vi "Get init instructions.vi"(8 "error in (no error)":errorcluster, 11 "Motor in":refnum<class "Motor.lvclass">) -> (0 "error out":errorcluster, 1 "name":string, 2 "init instructions":string[](array[string]), 3 "Motor out":refnum<class "Motor.lvclass">)   [LabVIEW 2018, in "Motor.lvclass"]
uses:
  Motor.lvclass
  Motor.lvclass/Motor.ctl
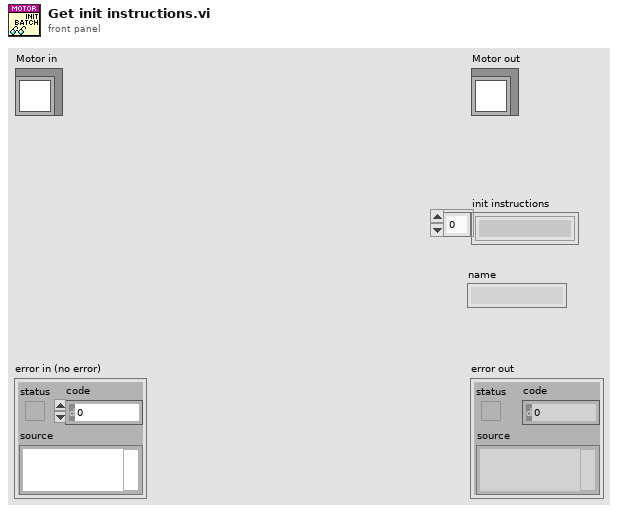
[diagram p1: front panel]
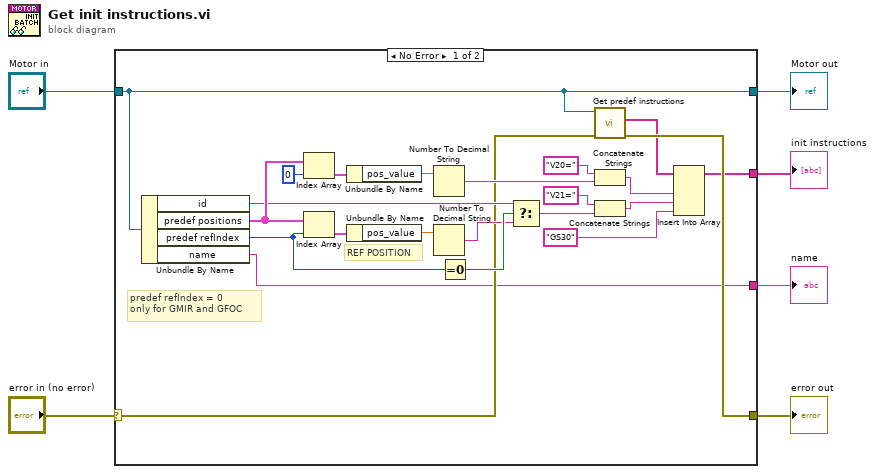
[diagram p0: block diagram]
diagram:
  n1 = case shown="No Error" "error in (no error)" {
    selector: "error in (no error)" -> [w14 w30]
    tunnel: [w13 w30] -> w5
    tunnel: [w15 w31] -> w3
    tunnel: "Motor in" -> [w15 w31]
    tunnel: [w12 _] -> w2
    tunnel: [w7 _] -> w1
    frame No Error {
      # "REF POSITION"
      # "predef refIndex = 0\nonly for GMIR and GFOC"
      n2 = Unbundle By Name(w15) -> ("id"=w20:string, "predef positions"=w25:cluster{"pos_name":string, "pos_value":dbl}[], "predef refIndex"=w27:i32, "name"=w7:string)
      n3 = Index Array(array=w25, index=0) -> (element=w26:cluster{"pos_name":string, "pos_value":dbl})
      n4 = Index Array(array=w25, index=w27) -> (element=w19:cluster{"pos_name":string, "pos_value":dbl})
      n5 = Unbundle By Name(w26) -> ("pos_value"=w23:dbl)
      n6 = Unbundle By Name(w19) -> ("pos_value"=w18:dbl)
      n7 = Number To Decimal String(number=w23) -> (decimal integer string=w22:string)  [unwired: 1 in]
      n8 = Number To Decimal String(number=w18) -> (decimal integer string=w17:string)  [unwired: 1 in]
      n9 = Equal To 0?(x=w27) -> (x = 0?=w21:bool)
      n10 = Select(t=w20, s=w21, f=w17) -> (s? t:f=w16:string)
      n11 = call-dynamic "Get predef instructions.vi"("error in (no error)"=w14, "Motor in"=w15) -> ("error out"=w13:errorcluster, "instructions"=w11:string[])  [unwired: 7 in, 1 out]
      n12 = Concatenate Strings("V20=" ("string"), w22) -> (w8:string)
      n13 = Concatenate Strings("V21=" ("string"), w16) -> (w9:string)
      n14 = Insert Into Array(array=w11, new element #1=w8, new element #2=w9, new element #3="GS30" ("string")) -> (w12:string[])  [unwired: 1 in]
    }
    frame Error {
    }
  }
  "error out" <- w5
  "Motor out" <- w3
  "init instructions" <- w2
  "name" <- w1
